vi "VerifConfigState.vi"(8 "error in (no error)":errorcluster, 11 "Acquisition in":refnum<class "Acquisition.lvclass">) -> (0 "error out":errorcluster, 3 "Acquisition out":refnum<class "Acquisition.lvclass">)   [LabVIEW 2018, in "Acquisition.lvclass"]
uses:
  Acquisition.lvclass
  Acquisition.lvclass/Acquisition.ctl
  Channel/Channel.lvclass
  StateMachine/State Machine.lvclass
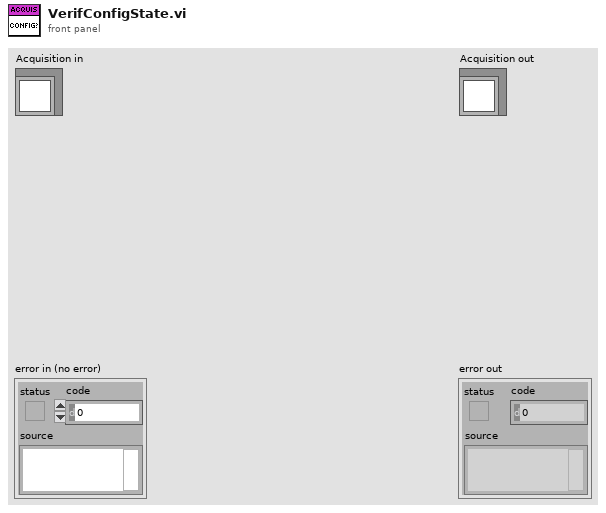
[diagram p1: front panel]
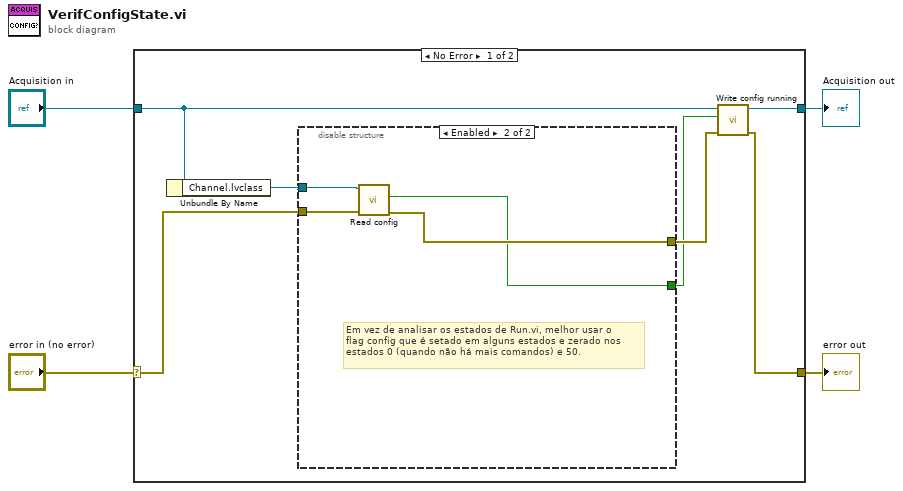
[diagram p0: block diagram]
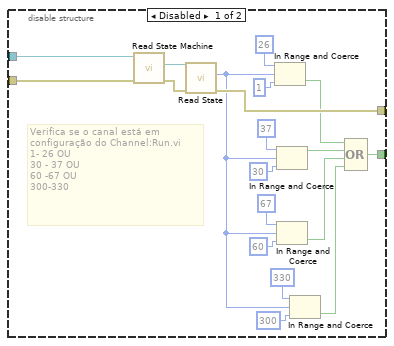
[diagram p2: hidden frame]
diagram:
  n1 = case shown="No Error" "error in (no error)" {
    selector: "error in (no error)" -> [w11 w36]
    tunnel: [w7 w36] -> w3
    tunnel: [w9 w35] -> w1
    tunnel: "Acquisition in" -> [w10 w35]
    frame No Error {
      n2 = Unbundle By Name(w10) -> ("Channel.lvclass"=w5:refnum<class "Channel.lvclass">)
      n3 = disable-structure shown="Enabled" {
        disable-tunnel: w11 -> [w27 w33]
        disable-tunnel: [w25 w32] -> w8
        disable-tunnel: [w17 w31] -> w6
        disable-tunnel: w5 -> [w12 w34]
        frame Disabled {
          # "Verifica se o canal está em \nconfiguração do Channel:Run.vi\n1- 26 OU\n30 - 37 OU\n60 -67 OU\n300-330"
          n4 = call-dynamic "Read State Machine.vi"("error in (no error)"=w27, "Device in"=w12) -> ("error out"=w26:errorcluster, "State Machine.lvclass"=w30:refnum<class "State Machine.lvclass">)  [unwired: 7 in, 1 out]
          n5 = call-dynamic "Read State.vi"("error in (no error)"=w26, "State Machine in"=w30) -> ("error out"=w25:errorcluster, "State"=w14:i32)  [unwired: 7 in, 1 out]
          n6 = In Range and Coerce(upper limit=26, x=w14, lower limit=1) -> (In Range?=w20:bool)  [unwired: 1 out]
          n7 = In Range and Coerce(upper limit=37, x=w14, lower limit=30) -> (In Range?=w19:bool)  [unwired: 1 out]
          n8 = In Range and Coerce(upper limit=67, x=w14, lower limit=60) -> (In Range?=w18:bool)  [unwired: 1 out]
          n9 = In Range and Coerce(upper limit=330, x=w14, lower limit=300) -> (In Range?=w13:bool)  [unwired: 1 out]
          n10 = Compound Arithmetic op=OR(w20, w19, w18, w13) -> (w17:bool)
        }
        frame Enabled {
          # "Em vez de analisar os estados de Run.vi, melhor usar o\nflag config que é setado em alguns estados e zerado nos\nestados 0 (quando não há mais comandos) e 50."
          n11 = call-dynamic "Read config.vi"("error in (no error)"=w33, "Channel in"=w34) -> ("error out"=w32:errorcluster, "config"=w31:bool)  [unwired: 7 in, 1 out]
        }
      }
      n12 = call-dynamic "Write config running.vi"("error in (no error)"=w8, "config running"=w6, "Server in"=w10) -> ("error out"=w7:errorcluster, "Server out"=w9:refnum<class "Acquisition.lvclass">)  [unwired: 7 in]
    }
    frame Error {
    }
  }
  "error out" <- w3
  "Acquisition out" <- w1
